vi "Resize.Resize Table within Tab Ctrl.vi"(5 "Pix from Bottom":i32, 6 "Min Size":cluster{"Width":i32, "Height":i32}={"Width"=250, "Height"=200}, 7 "Pix from Right":i32, 8 "error in":errorcluster, 9 "Aspect Ratio":cluster{"W/H":dbl, "Enable":bool}={"W/H"=1.0, "Enable"=FALSE} {"W/H" format="%.2g"}, 10 "Table Ctrl":refnum<vi>, 11 "Tab Ctrl":refnum<vi>) -> (0 "error out":errorcluster, 2 "Table Ctrl Out":refnum<vi>, 3 "Tab Ctrl Out":refnum<vi>)   [LabVIEW 2024, in "EQMF.lvlib" / "Controls.lvlib"]
uses:
  Controls.lvlib
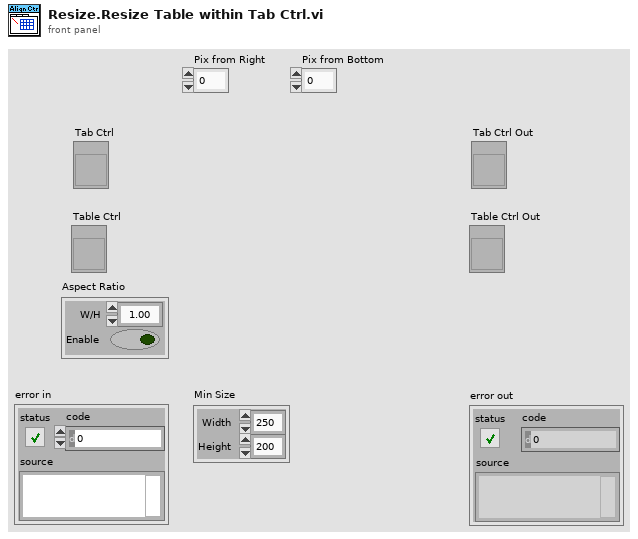
[diagram p1: front panel]
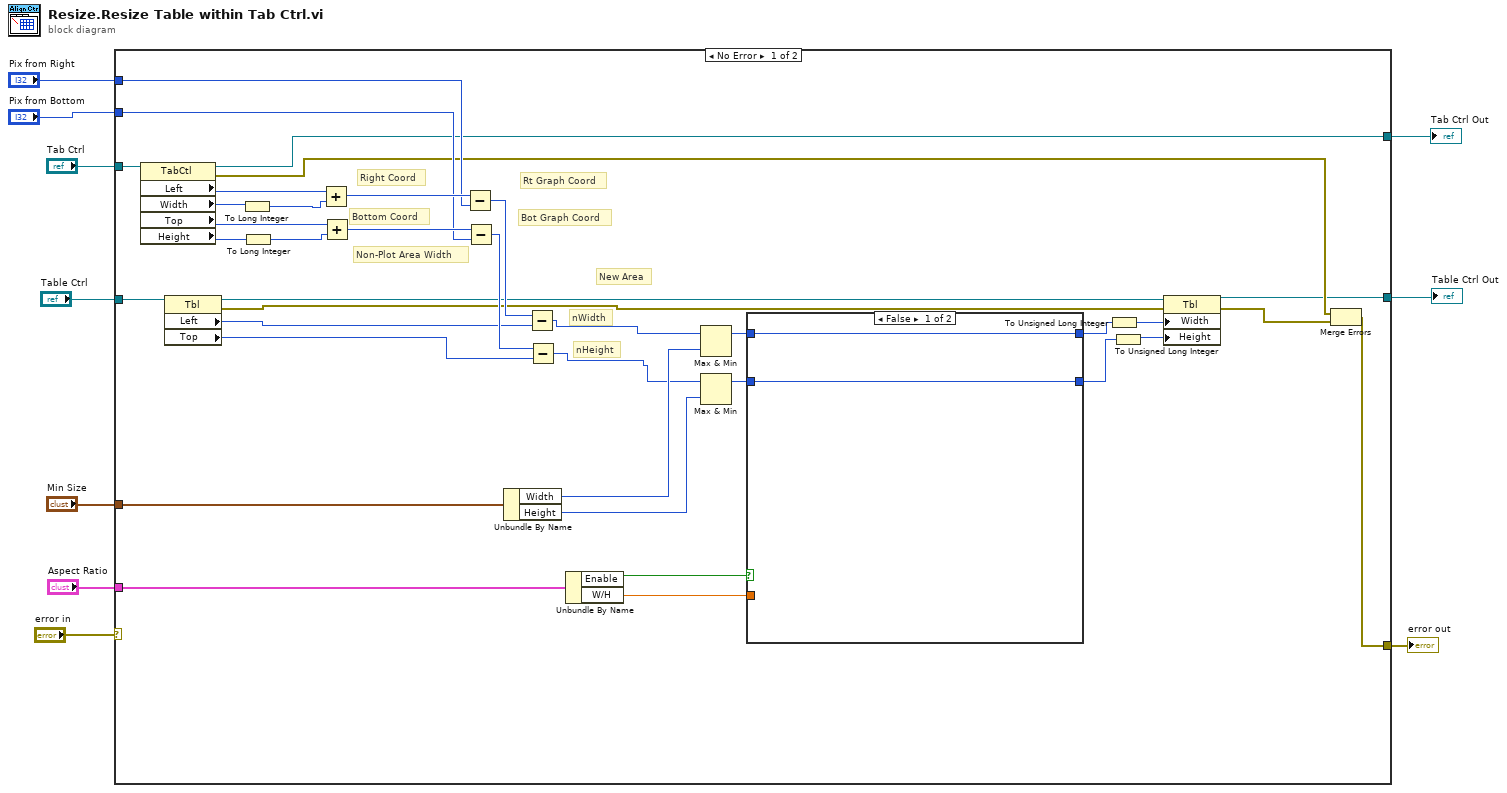
[diagram p0: block diagram]
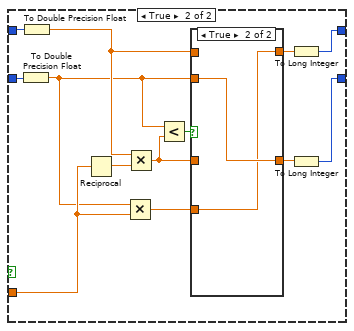
[diagram p2: hidden frame]
diagram:
  n1 = case shown="No Error" "error in" {
    selector: "error in" -> [_ w67]
    tunnel: "Pix from Right" -> [w39 _]
    tunnel: "Pix from Bottom" -> [w38 _]
    tunnel: [w31 w67] -> w8
    tunnel: "Min Size" -> [w30 _]
    tunnel: "Aspect Ratio" -> [w25 _]
    tunnel: "Tab Ctrl" -> [w22 w69]
    tunnel: "Table Ctrl" -> [w21 w68]
    tunnel: [w18 w69] -> w3
    tunnel: [w17 w68] -> w2
    frame No Error {
      # "nHeight"
      # "nWidth"
      # "New Area"
      # "Bot Graph Coord"
      # "Rt Graph Coord"
      # "Non-Plot Area Width"
      # "Bottom Coord"
      # "Right Coord"
      n2 = property on="Property Node" class="TabCtl"(reference=w22) -> (reference out=w18:refnum<vi>, error out=w20:errorcluster, "Left"=w42:i32, "Width"=w45:u32, "Top"=w43:i32, "Height"=w44:u32)  [unwired: 1 in]
      n3 = property on="Property Node" class="Tbl"(reference=w21) -> (reference out=w33:refnum<vi>, error out=w32:errorcluster, "Left"=w35:i32, "Top"=w34:i32)  [unwired: 1 in]
      n4 = To Long Integer(number=w45) -> (32bit integer=w46:i32)
      n5 = To Long Integer(number=w44) -> (32bit integer=w47:i32)
      n6 = Add(x=w42, y=w46) -> (x+y=w40:i32)
      n7 = Add(x=w43, y=w47) -> (x+y=w41:i32)
      n8 = Subtract(x=w40, y=w39) -> (x-y=w37:i32)
      n9 = Subtract(x=w41, y=w38) -> (x-y=w36:i32)
      n10 = Unbundle By Name(w30) -> ("Width"=w29:i32, "Height"=w28:i32)
      n11 = Subtract(x=w37, y=w35) -> (x-y=w12:i32)
      n12 = Subtract(x=w36, y=w34) -> (x-y=w11:i32)
      n13 = Unbundle By Name(w25) -> ("Enable"=w24:bool, "W/H"=w23:dbl)
      n14 = Max & Min(x=w12, y=w29) -> (max(x,y)=w27:i32)  [unwired: 1 out]
      n15 = Max & Min(x=w11, y=w28) -> (max(x,y)=w26:i32)  [unwired: 1 out]
      n16 = case shown="False" w24 {
        tunnel: w27 -> [w49 w62]
        tunnel: w26 -> [w48 w61]
        tunnel: [w49 w53] -> w13
        tunnel: [w48 w54] -> w14
        tunnel: w23 -> [_ w59]
        frame False {
        }
        frame True {
          n17 = To Double Precision Float(number=w61) -> (double precision float=w51:dbl)
          n18 = To Double Precision Float(number=w62) -> (double precision float=w58:dbl)
          n19 = Reciprocal(x=w59) -> (1/x=w60:dbl)
          n20 = Multiply(x=w51, y=w59) -> (x*y=w50:dbl)
          n21 = Multiply(x=w58, y=w60) -> (x*y=w57:dbl)
          n22 = Less?(x=w51, y=w57) -> (x < y?=w56:bool)
          n23 = case shown="True" w56 {
            tunnel: w58 -> [w64 _]
            tunnel: w57 -> [w63 _]
            tunnel: [w64 w65] -> w52
            tunnel: [w63 w66] -> w55
            tunnel: w51 -> [_ w66]
            tunnel: w50 -> [_ w65]
            frame False {
            }
            frame True {
            }
          }
          n24 = To Long Integer(number=w52) -> (32bit integer=w53:i32)
          n25 = To Long Integer(number=w55) -> (32bit integer=w54:i32)
        }
      }
      n26 = To Unsigned Long Integer(number=w13) -> (unsigned 32bit integer=w16:u32)
      n27 = To Unsigned Long Integer(number=w14) -> (unsigned 32bit integer=w15:u32)
      n28 = property on="Property Node" class="Tbl"(reference=w33, error in=w32, "Width"=w16, "Height"=w15) -> (reference out=w17:refnum<vi>, error out=w19:errorcluster)
      n29 = Merge Errors(w20, w19) -> (w31:errorcluster)
    }
    frame Error {
    }
  }
  "error out" <- w8
  "Tab Ctrl Out" <- w3
  "Table Ctrl Out" <- w2
